vi "Spread Fire.vi"(9 "Pixel Source":i32, 10 "Width":i32, 11 "Pixel Array In":i32[](array[numeric])) -> (3 "Pixel Array Out":i32[](array[numeric]))   [LabVIEW 2018]
doc: "This is the core of the fire effect, and randomly moves each fire pixel upward while decreasing its intensity (from white hot through the palette to black)."
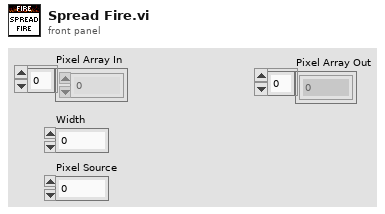
[diagram p1: front panel]
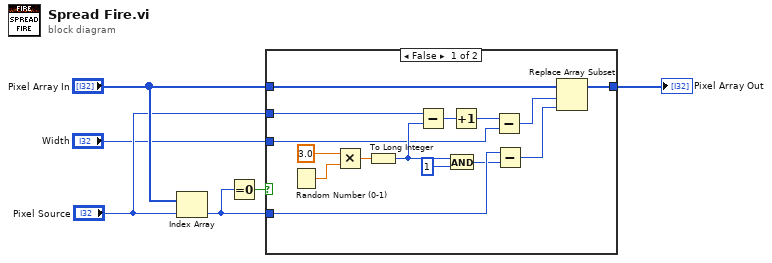
[diagram p0: block diagram]
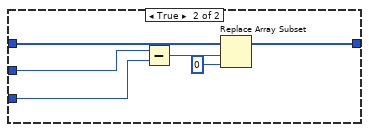
[diagram p2: hidden frame]
diagram:
  n1 = Index Array(array="Pixel Array In", index="Pixel Source") -> (element=w5:i32)
  n2 = Equal To 0?(x=w5) -> (x = 0?=w6:bool)
  n3 = case shown="False" w6 {
    tunnel: "Pixel Array In" -> [w16 w27]
    tunnel: "Pixel Source" -> [w18 w26]
    tunnel: [w15 w23] -> w3
    tunnel: w5 -> [w12 _]
    tunnel: "Width" -> [w7 w22]
    frame False {
      n4 = Random Number (0-1)() -> (number: 0 to 1=w21:dbl)
      n5 = Multiply(x=3.0 ("y"), y=w21) -> (x*y=w19:dbl)
      n6 = To Long Integer(number=w19) -> (32bit integer=w11:i32)
      n7 = Subtract(x=w18, y=w11) -> (x-y=w17:i32)
      n8 = And(x=w11, y=1) -> (x .and. y?=w9:i32)
      n9 = Increment(x=w17) -> (x+1=w14:i32)
      n10 = Subtract(x=w14, y=w7) -> (x-y=w13:i32)
      n11 = Subtract(x=w12, y=w9) -> (x-y=w8:i32)
      n12 = Replace Array Subset(array=w16, new element=w8, index=w13) -> (w15:i32[])
    }
    frame True {
      n13 = Subtract(x=w26, y=w22) -> (x-y=w25:i32)
      n14 = Replace Array Subset(array=w27, new element=0 ("new element/subarray"), index=w25) -> (w23:i32[])
    }
  }
  "Pixel Array Out" <- w3
